vi "Get External Trigger Termination.vi"(8 "error in (no error)":errorcluster, 11 "puiTermination":u32) -> (0 "error out":errorcluster, 2 "function return":u32, 3 "puiTermination out":u32)   [LabVIEW 2014, in "atmcd32d.lvlib"]
doc: "unsigned int WINAPI GetExternalTriggerTermination(at_u32 * puiTermination);"
uses:
  atmcd32d.lvlib
  atmcd32d.dll
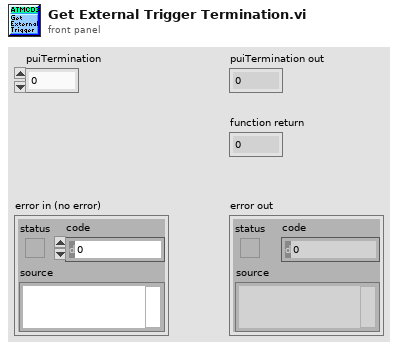
[diagram p1: front panel]
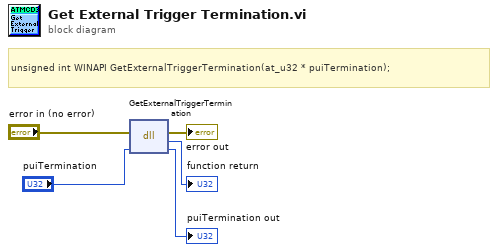
[diagram p0: block diagram]
diagram:
  # "unsigned int WINAPI GetExternalTriggerTermination(at_u32 * puiTermination);"
  n1 = dll-call lib="C:/Users/Bakir/Documents/Lambda2-Testing/lib/Andorlib/atmcd32d.*" fn="GetExternalTriggerTermination"(error in="error in (no error)", "puiTermination"="puiTermination") -> (error out=→"error out":errorcluster, →"function return":u32, "puiTermination"=→"puiTermination out":u32)  [unwired: 2 in, 1 out]
